vi "To bytes.vi"(11 "MessagePackNumeric in":refnum<class "MessagePackNumeric.lvclass">) -> (2 "Array":u8[](array[numeric]), 3 "MessagePackNumeric out":refnum<class "MessagePackNumeric.lvclass">)   [LabVIEW 2020, in "MessagePack.lvlib" / "MessagePackNumeric.lvclass"]
uses:
  MessagePackNumeric.lvclass
  MessagePackNumeric.lvclass/MessagePackNumeric.ctl
  MessagePack.lvlib
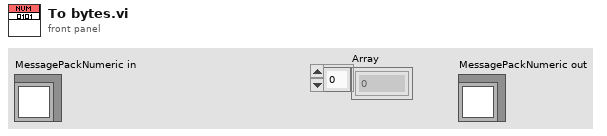
[diagram p1: front panel]
types:
  T1 = typedef "MessagePack.lvlib/MsgPack Object Types.ctl" = enum16{"UNSUPPORTED", "POSINT", "NEGINT", "FIXMAP", "FIXARRAY", "FIXSTR", "NIL", "FALSE", "TRUE", "BIN8", "BIN16", "BIN32", "EXT8", "EXT16", "EXT32", "FLOAT32", "FLOAT64", "UINT8", "UINT16", "UINT32", "UINT64", "INT8", "INT16", "INT32", "INT64", "FIXEXT1", "FIXEXT2", "FIXEXT4", "FIXEXT8", "FIXEXT16", "STR8", "STR16", "STR32", "ARRAY16", "ARRAY32", "MAP16", "MAP32"}
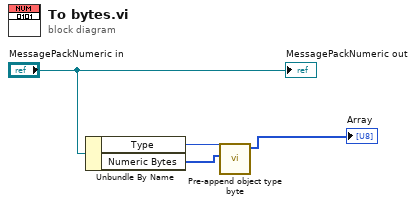
[diagram p0: block diagram]
diagram:
  n1 = Unbundle By Name("MessagePackNumeric in") -> ("Type"=w3:T1, "Numeric Bytes"=w2:u8[])
  n2 = call "Pre-append object type byte.vi"("bytes in"=w2, "Object type"=w3) -> ("encoded bytes"=→"Array":u8[])  [unwired: 8 in, 1 out]
  "MessagePackNumeric out" <- "MessagePackNumeric in"
